vi "PalmSense Configure CP.vi"(8 "error in (no error)":errorcluster, 10 "Message Data":variant, 11 "Data Cluster in":T1) -> (0 "error out":errorcluster, 3 "Data Cluster out":T1)   [LabVIEW 2020, in "PalmSens.lvlib"]
uses:
  PalmSens.lvlib
  PalmSense Hardware Configuration.ctl
  <instrlib>/PalmSens SDK for LabVIEW 5.10/PalmSens/PalmSens.lvclass
  support/Message Queue/Message Cluster.ctl
  support/HW Message Cluster.ctl
  C:/Program Files (x86)/National Instruments/LabVIEW 2020/instr.lib/PalmSens SDK for LabVIEW 5.10/PalmSens/Libraries/PalmSens.Core.dll
  support/Message Queue/Message Queue.lvlib
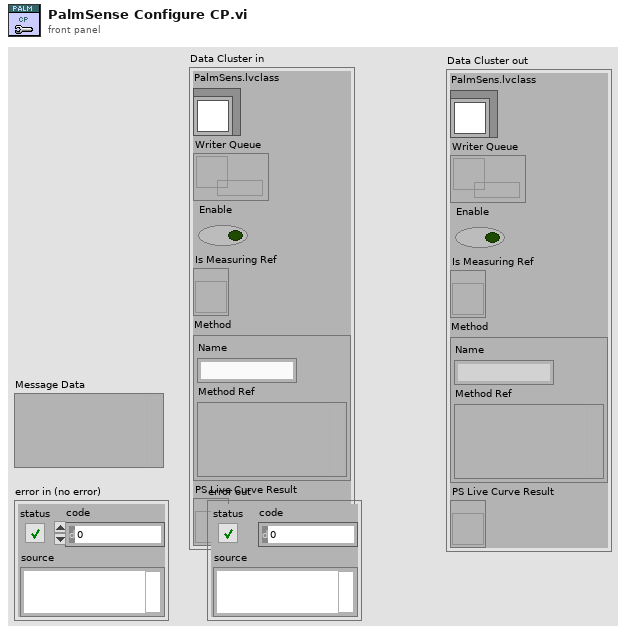
[diagram p1: front panel]
types:
  T1 = typedef "PalmSens.lvlib/PalmSense Hardware Configuration.ctl" = cluster{"PalmSens.lvclass":refnum<class "PalmSens.lvclass">, "Writer Queue":refnum<queue>, "Enable":bool, "Is Measuring Ref":refnum<vi>, "Method":cluster{"Name":string, "Method Ref":variant}, "PS Live Curve Result":refnum<vi>}
  T2 = cluster{"Current":dbl, "IntervalTime":dbl, "RunTime":dbl}
  T3 = typedef "Message Queue.lvlib/HW Message Cluster.ctl" = cluster{"Writer Queue":refnum<queue>, "Writer Data":T4}
  T4 = typedef "Message Queue.lvlib/Message Cluster.ctl" = cluster{"Message":string, "Message Data":variant}
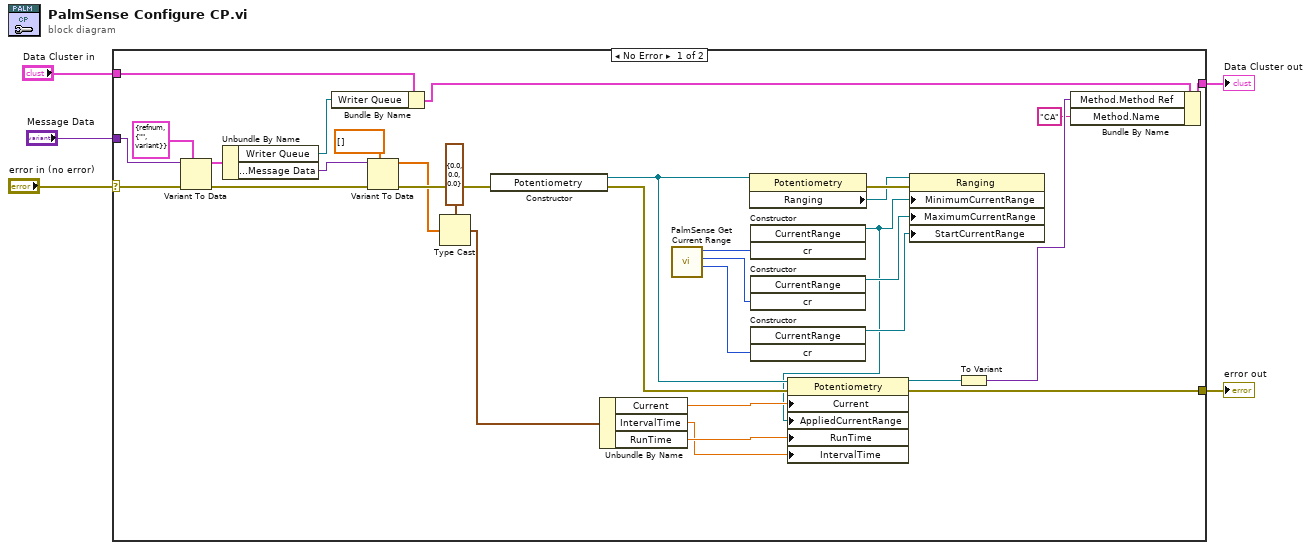
[diagram p0: block diagram]
diagram:
  n1 = case shown="No Error" "error in (no error)" {
    selector: "error in (no error)" -> [w34 w38]
    tunnel: "Message Data" -> [w32 _]
    tunnel: [w19 w39] -> w4
    tunnel: "Data Cluster in" -> [w36 w39]
    tunnel: [w22 w38] -> w2
    frame No Error {
      n2 = Variant To Data(error in=w34, type=T3 {"Writer Queue"=refnum, "Writer Data"={"Message"="", "Message Data"=variant}}, Variant=w32) -> (data=w35:T3, error out=w33:errorcluster)
      n3 = Unbundle By Name(w35) -> ("Writer Queue"=w30:refnum<queue>, "Writer Data.Message Data"=w31:variant)
      n4 = Bundle By Name(cluster=w36, "Writer Queue"=w30) -> (w37:T1)
      n5 = Variant To Data(error in=w33, type=dbl[] [] ("LSV Scan"), Variant=w31) -> (data=w14:dbl[], error out=w28:errorcluster)
      n6 = Type Cast(type=T2 {"Current"=0.0, "IntervalTime"=0.0, "RunTime"=0.0} ("cluster"), x=w14) -> (*(type *) &x=w12:T2)
      n7 = constructor class="Potentiometry"(error in=w28) -> (reference out=w26:refnum<k24>, error out=w27:errorcluster)  [unwired: 2 in, 1 out]
      n8 = Unbundle By Name(w12) -> ("Current"=w23:dbl, "IntervalTime"=w10:dbl, "RunTime"=w11:dbl)
      n9 = call "PalmSense Get Current Range.vi"() -> ("Start Current Range"=w8:i32, "Max Current Range"=w7:i32, "Min Current Range"=w6:i32)  [unwired: 9 in]
      n10 = property class="Potentiometry"(reference=w26) -> (error out=w25:errorcluster, "Ranging"=w24:refnum<k24>)  [unwired: 1 in, 1 out]
      n11 = constructor class="CurrentRange"("cr"=w6) -> (reference out=w9:refnum<k24>)  [unwired: 3 in, 3 out]
      n12 = constructor class="CurrentRange"("cr"=w7) -> (reference out=w21:refnum<k24>)  [unwired: 3 in, 3 out]
      n13 = constructor class="CurrentRange"("cr"=w8) -> (reference out=w20:refnum<k24>)  [unwired: 3 in, 3 out]
      n14 = property class="Potentiometry"(reference=w26, error in=w27, "Current"=w23, "AppliedCurrentRange"=w9, "RunTime"=w11, "IntervalTime"=w10) -> (reference out=w18:refnum<k24>, error out=w22:errorcluster)
      n15 = property class="Ranging"(reference=w24, error in=w25, "MinimumCurrentRange"=w9, "MaximumCurrentRange"=w21, "StartCurrentRange"=w20) -> ()  [unwired: 2 out]
      n16 = To Variant(anything=w18) -> (Variant=w17:variant)
      n17 = Bundle By Name(cluster=w37, "Method.Method Ref"=w17, "Method.Name"="CA") -> (w19:T1)
    }
    frame Error {
    }
  }
  "Data Cluster out" <- w4
  "error out" <- w2
